vi "Get file group chan waveform.vi"(6 "Clear missing ch err":bool=TRUE, 7 "Clip/desimate":T1={"Clip time"=FALSE, "Tiime 0"=0.0, "Time 1"=0.0, "Maximum data points"=-1, "Decimation method"=enum."Min-Max"}, 8 "Error In":errorcluster, 9 "Channel":string, 10 "Group":string, 11 "File":path) -> (0 "Error Out":errorcluster, 2 "Valid WFRM":bool, 3 "Waveform":waveform(sgl))   [LabVIEW 2018]
uses:
  Controls/Data reduction.ctl
  577bf0d0-391d-4339-897f-1f744d455536.vi
  <vilib>/Utility/error.llb/Clear Errors.vi
  <vilib>/ErrorRing/Error Ring.xnode
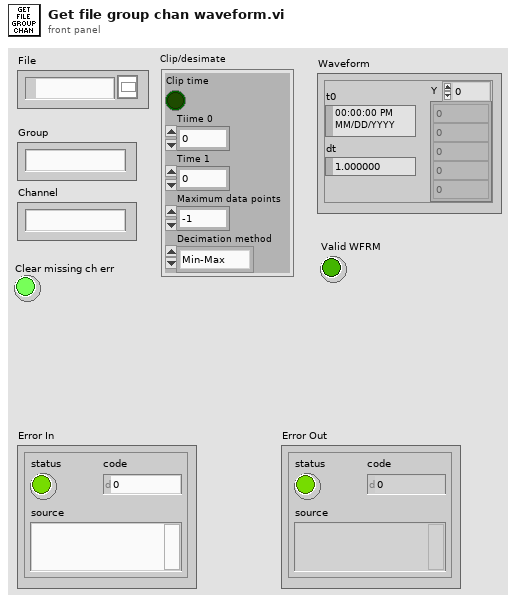
[diagram p1: front panel]
types:
  T1 = typedef "Data reduction.ctl" = cluster{"Clip time":bool, "Tiime 0":dbl, "Time 1":dbl, "Maximum data points":i32, "Decimation method":enum16{"coerce", "linear", "spline", "Min-Max", "Average"}}
  T2 = enum16{"open", "open or create", "create or replace", "create", "open (read-only)"}
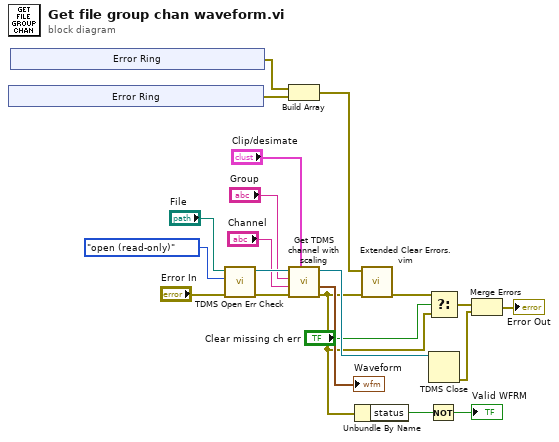
[diagram p0: block diagram]
diagram:
  n1 = xnode "Error Ring"() -> ("error out"=w3:errorcluster)
  n2 = xnode "Error Ring"() -> ("error out"=w4:errorcluster)
  n3 = call "TDMS Open Err Check.vi"("Error In"="Error In", "operation (0:open)"=T2."open (read-only)", "File Path Control"="File") -> ("Error Out"=w15:errorcluster, "tdms file out"=w17:refnum<k34>)  [unwired: 6 in, 1 out]
  n4 = Build Array(w4, w3) -> (w1:errorcluster[])
  n5 = call "Get TDMS channel with scaling.vi"("Clip/desimate"="Clip/desimate", "error in"=w15, "Channel name"="Channel", "group name"="Group", "tdms file"=w17) -> ("error out"=w7:errorcluster, "output waveform"=→"Waveform":waveform(sgl), "tdms file out"=w16:refnum<k34>)  [unwired: 4 in]
  n6 = Unbundle By Name(w7) -> ("status"=w9:bool)
  n7 = call "Extended Clear Errors.vim"("Error In"=w7, "specific error code to clear (0: all)"=w1) -> ("Error Out"=w2:errorcluster)  [unwired: 7 in, 2 out]
  n8 = Not(x=w9) -> (.not. x?=→"Valid WFRM":bool)
  n9 = Select(t=w2, s="Clear missing ch err", f=w7) -> (s? t:f=w6:errorcluster)
  n10 = TDMS Close(11:w16) -> (0:w20:errorcluster)  [unwired: 1 in, 1 out]
  n11 = Merge Errors(w6, w20) -> (→"Error Out":errorcluster)
